vi "hidSPD Read Report.vi"(8 "error in (no error)":errorcluster, 11 "spdDevSession in":T1) -> (0 "error out":errorcluster, 2 "hidSPD Simple Report":T2, 3 "spdDevSession out":T1)   [LabVIEW 2018, in "hidSPDLibForLabView.lvlib"]
uses:
  hidSPDLibForLabView.lvlib
  hidSPD Controls/hidSPD Simple Report.ctl
  hidSPD Controls/hidSPD Device Session.ctl
  <vilib>/Utility/error.llb/Error Cluster From Error Code.vi
  <vilib>/ErrorRing/Error Ring.xnode
  hidSPD DLL files/libSPD.dll
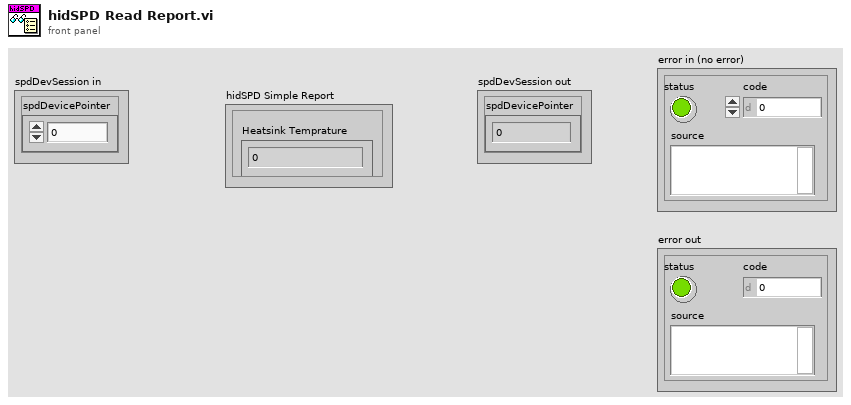
[diagram p1: front panel]
types:
  T1 = typedef "hidSPDLibForLabView.lvlib/hidSPD Device Session.ctl" = cluster{"spdDevicePointer":u64}
  T2 = typedef "hidSPDLibForLabView.lvlib/hidSPD Simple Report.ctl" = cluster{"Heatsink Temprature":sgl, "Diod Temprature":sgl, "TEC-voltage":sgl, "Diod Bias":sgl, "RF Power":sgl, "Thermal used":sgl, "hv bias used":sgl, "hv code used":u16, "strobe code used":u16, "SPD number":u8, "SPD ready":u8}
  T3 = enum16{"big-endian, network order", "native, host order", "little-endian"}
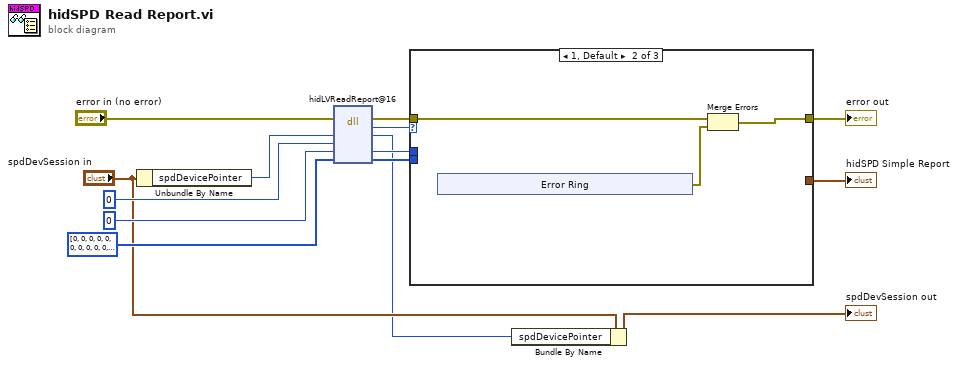
[diagram p0: block diagram]
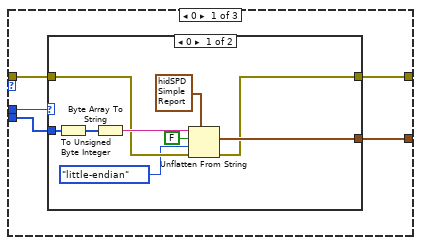
[diagram p2: hidden frame]
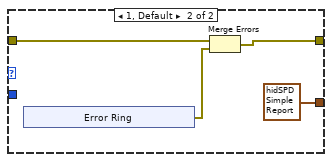
[diagram p3: hidden frame]
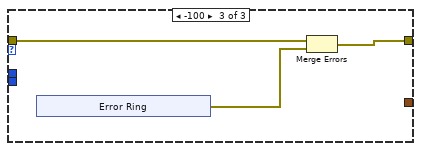
[diagram p4: hidden frame]
diagram:
  n1 = Unbundle By Name("spdDevSession in") -> ("spdDevicePointer"=w4:u64)
  n2 = dll-call lib="D:/NextCloud/SPD/hidSPDLibForLabView/hidSPD DLL files/libSPD.dll" fn="hidLVReadReport@16"(error in="error in (no error)", "spdDeviceHandle"=w4, "id"=0 ("report"), "cmd"=0, "data"=i32[] [0, 0, 0, 0, 0, 0, 0, 0, 0, 0, 0, 0, 0, 0, 0, 0, 0, 0, 0, 0, 0, 0, 0, 0, 0, 0, 0, 0, 0, 0, 0, 0, 0, 0, 0, 0, 0, 0, 0, 0, 0, 0, 0, 0, 0, 0, 0, 0, 0, 0, 0, 0, 0, 0, 0, 0, 0, 0, 0, 0, 0, 0]) -> (error out=w5:errorcluster, "error"=w6:i32, "spdDeviceHandle"=w2:u64, "cmd"=w7:i32, "data"=w8:i32[])  [unwired: 3 in, 1 out]
  n3 = case shown="1, Default" w6 {
    tunnel: [w19 w38 w46] -> w14
    tunnel: [w18 _ _] -> w13
    tunnel: w8 -> [w17 _ _]
    tunnel: w7 -> [w16 _ _]
    tunnel: w5 -> [w15 w40 w48]
    frame 0 {
      n4 = case shown="0" w16 {
        tunnel: w17 -> [w28 _]
        tunnel: w15 -> [w24 w32]
        tunnel: [w22 w30] -> w19
        tunnel: [w23 T2 {"Heatsink Temprature"=0.0, "Diod Temprature"=0.0, "TEC-voltage"=0.0, "Diod Bias"=0.0, "RF Power"=0.0, "Thermal used"=0.0, "hv bias used"=0.0, "hv code used"=0, "strobe code used"=0, "SPD number"=0, "SPD ready"=0} ("hidSPD Simple Report")] -> w18
        frame 0 {
          n5 = To Unsigned Byte Integer(number=w28) -> (unsigned 8bit integer=w27:u8[])
          n6 = Byte Array To String(unsigned byte array=w27) -> (string=w26:string)
          n7 = Unflatten From String(type=T2 {"Heatsink Temprature"=0.0, "Diod Temprature"=0.0, "TEC-voltage"=0.0, "Diod Bias"=0.0, "RF Power"=0.0, "Thermal used"=0.0, "hv bias used"=0.0, "hv code used"=0, "strobe code used"=0, "SPD number"=0, "SPD ready"=0} ("hidSPD Simple Report"), binary string=w26, data includes array or string size? (T)=FALSE, byte order (0:big-endian, network order)=T3."little-endian", error in (no error)=w24) -> (value=w23:T2, error out=w22:errorcluster)  [unwired: 1 out]
        }
        frame 1, Default {
          n8 = xnode "Error Ring"() -> ("error out"=w31:errorcluster)
          n9 = Merge Errors(w32, w31) -> (w30:errorcluster)
        }
      }
    }
    frame 1, Default {
      n10 = xnode "Error Ring"() -> ("error out"=w39:errorcluster)
      n11 = Merge Errors(w40, w39) -> (w38:errorcluster)
    }
    frame -100 {
      n12 = xnode "Error Ring"() -> ("error out"=w47:errorcluster)
      n13 = Merge Errors(w48, w47) -> (w46:errorcluster)
    }
  }
  "error out" <- w14
  "hidSPD Simple Report" <- w13
  n14 = Bundle By Name(cluster="spdDevSession in", "spdDevicePointer"=w2) -> (→"spdDevSession out":T1)
